vi "Get_Meas_Mode.vi"(2 "error in (no error)":errorcluster, 4 "VISA in":refnum<visa-resource-name>) -> (0 "error out":errorcluster, 1 "VISA out":refnum<visa-resource-name>, 3 "Measurement mode":enum16{"MODE 1", "MODE 2", "UNKNOWN"}(ring))   [LabVIEW 2017, in "GP22_TDC_Arduinoed.lvlib"]
doc: "Set the GP22's internal registers to the given values. \n/* NOT IMPLEMENTED YET - If an input value of \"-1\" is given, the subVI will use ACAM's default settings for that register instead. */"
uses:
  <vilib>/regexp/Match Regular Expression.xnode
  GP22_TDC_Arduinoed.lvlib
panel:
  out "read buffer":string
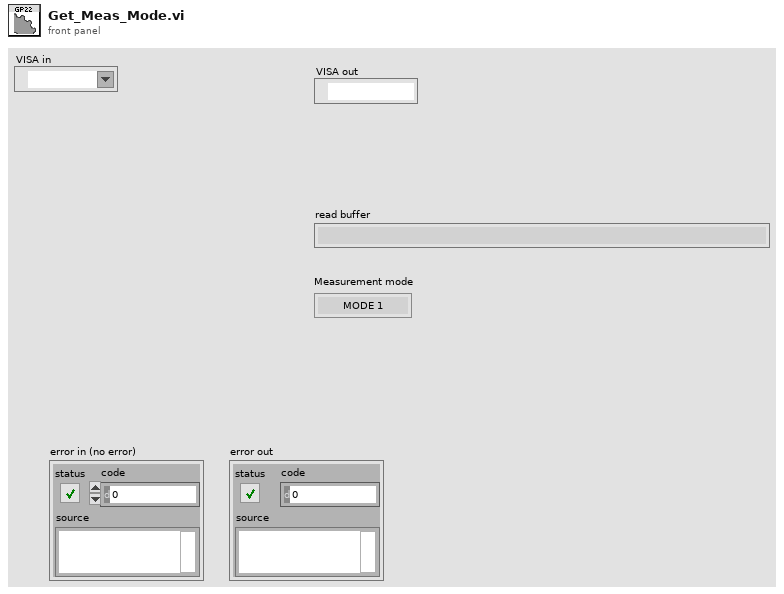
[diagram p1: front panel]
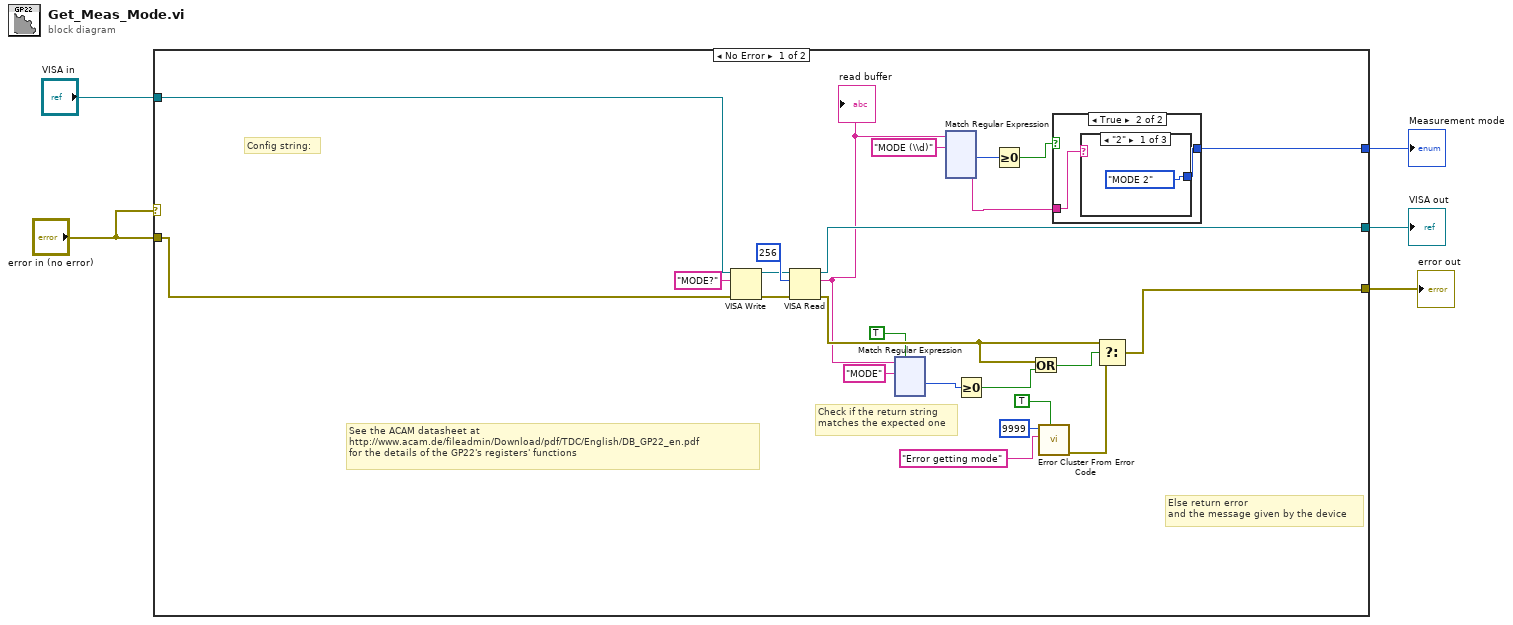
[diagram p0: block diagram]
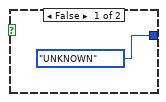
[diagram p2: hidden frame]
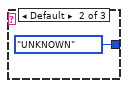
[diagram p3: hidden frame]
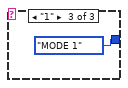
[diagram p4: hidden frame]
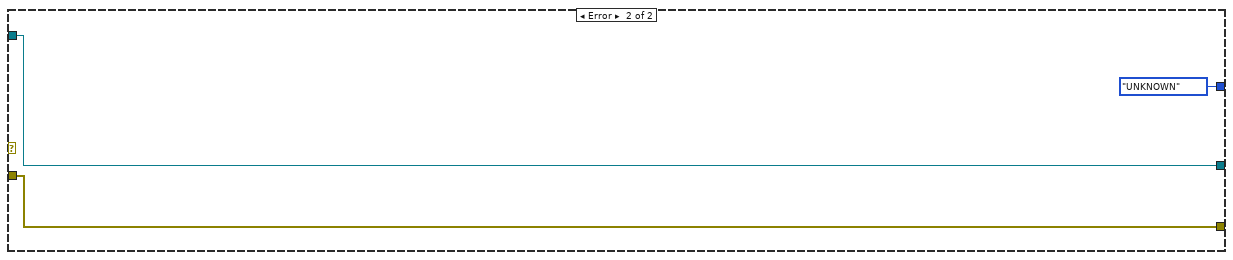
[diagram p5: hidden frame]
diagram:
  n1 = case shown="No Error" "error in (no error)" {
    tunnel: [w29 w268] -> w5
    tunnel: "error in (no error)" -> [w21 w268]
    tunnel: [w23 w267] -> w3
    tunnel: "VISA in" -> [w22 w267]
    tunnel: [w6 enum16{"MODE 1", "MODE 2", "UNKNOWN"}."UNKNOWN" ("Measurement mode")] -> w1
    frame No Error {
      # "See the ACAM datasheet at \nhttp://www.acam.de/fileadmin/Download/pdf/TDC/English/DB_GP22_en.pdf\nfor the details of the GP22's registers' functions"
      # "Config string:"
      # "Else return error\nand the message given by the device"
      # "Check if the return string\nmatches the expected one"
      n2 = VISA Write(VISA resource name=w22, write buffer="MODE?", error in (no error)=w21) -> (VISA resource name out=w26:refnum<visa-resource-name>, error out=w27:errorcluster)  [unwired: 1 out]
      n3 = VISA Read(VISA resource name=w26, byte count=u32 256, error in (no error)=w27) -> (VISA resource name out=w23:refnum<visa-resource-name>, read buffer=w11:string, error out=w25:errorcluster)  [unwired: 1 out]
      "read buffer" <- w11
      n4 = xnode "Match Regular Expression"("input string"=w11, "regular expression"="MODE", "ignore case? (F)"=TRUE) -> ("offset past match"=w19:i32)  [unwired: 3 in, 4 out]
      n5 = xnode "Match Regular Expression"("input string"=w11, "regular expression"="MODE (\\d)") -> ("offset past match"=w9:i32, "submatch 1"=w7:string)  [unwired: 4 in, 4 out]
      n6 = Greater Or Equal To 0?(x=w19) -> (x >= 0?=w14:bool)
      n7 = Greater Or Equal To 0?(x=w9) -> (x >= 0?=w8:bool)
      n8 = Or(x=w25, y=w14) -> (x .or. y?=w24:bool)
      n9 = call <vilib>:"Error Cluster From Error Code.vi"("show call chain? (False)"=TRUE, "error message (\"\")"="Error getting mode" ("string"), "error code (0)"=9999) -> ("error out"=w15:errorcluster)  [unwired: 6 in]
      n10 = case shown="True" w8 {
        tunnel: w7 -> [_ w32]
        tunnel: [enum16{"MODE 1", "MODE 2", "UNKNOWN"}."UNKNOWN" ("Measurement mode") w31] -> w6
        frame False {
        }
        frame True {
          n11 = case shown="\"2\"" w32 {
            tunnel: [enum16{"MODE 1", "MODE 2", "UNKNOWN"}."MODE 2" ("Measurement mode") enum16{"MODE 1", "MODE 2", "UNKNOWN"}."UNKNOWN" ("Measurement mode") enum16{"MODE 1", "MODE 2", "UNKNOWN"}."MODE 1" ("Measurement mode")] -> w31
            frame "2" {
            }
            frame Default {
            }
            frame "1" {
            }
          }
        }
      }
      n12 = Select(t=w25, s=w24, f=w15) -> (s? t:f=w29:errorcluster)
    }
    frame Error {
    }
  }
  "error out" <- w5
  "VISA out" <- w3
  "Measurement mode" <- w1
